vi "gfitsio-read-image-subset-i32-2d.vi"(4 "lpixel (-1,-1: rest)":cluster{"X":i32, "Y":i32}={"X"=-1, "Y"=-1}, 6 "fpixel (1,1)":cluster{"X":i32, "Y":i32}={"X"=1, "Y"=1}, 7 "inc (1,1)":cluster{"X":i32, "Y":i32}={"X"=1, "Y"=1}, 8 "error in (no error)":errorcluster, 9 "nulval (0: don't check)":i32, 11 "gfits refnum":T1) -> (0 "error out":errorcluster, 1 "anynul":bool, 2 "data":i32[][](array[numeric]), 3 "dup gfits refnum":T1)   [LabVIEW 2019, in "gfitsio.lvlib"]
doc: "Read a rectangular subimage (or the whole image) from the FITS data array. <B>fpixel</B> and <B>lpixel</B> give the coordinates of the first (lower left corner) and last (upper right corner) pixels to be read from the FITS image. Undefined FITS array elements will be set equal to <B>nullval</B> unless <B>nulval</B> is zero in which case no checks for undefined pixels will be performed."
uses:
  gfitsio.lvlib
  gfitsio-refnum.ctl
  cfitsio-hdutypes.ctl
  gfitsio.dll
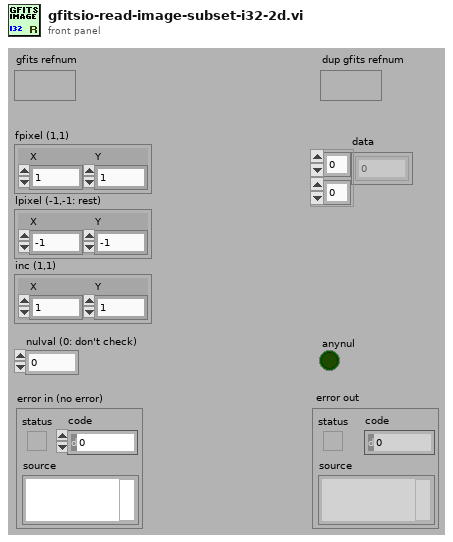
[diagram p1: front panel]
types:
  T1 = typedef "gfitsio.lvlib/gfitsio-refnum.ctl" = refnum<k1>
  T2 = typedef "gfitsio.lvlib/cfitsio-hdutypes.ctl" = i32
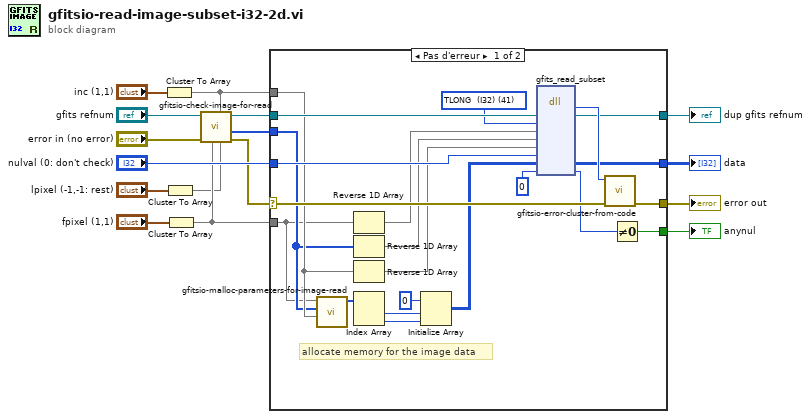
[diagram p0: block diagram]
diagram:
  n1 = Cluster To Array(cluster="inc (1,1)") -> (array=w1:i32[])
  n2 = Cluster To Array(cluster="lpixel (-1,-1: rest)") -> (array=w2:i32[])
  n3 = Cluster To Array(cluster="fpixel (1,1)") -> (array=w3:i32[])
  n4 = call "gfitsio-check-image-for-read.vi"("lpixel"=w2, "inc"=w1, "fpixel"=w3, "error in (no error)"="error in (no error)", "gfits refnum"="gfits refnum") -> ("error out"=w5:errorcluster, "lpixel out"=w4:i32[], "dup gfits refnum"=w10:T1)  [unwired: 4 in]
  n5 = case shown="Pas d'erreur" w5 {
    selector: w5 -> [w33 w39]
    tunnel: [w37 w39] -> w15
    tunnel: w10 -> [w35 w40]
    tunnel: [w34 w40] -> w16
    tunnel: "nulval (0: don't check)" -> [w32 _]
    tunnel: [w30 _] -> w13
    tunnel: [w29 _] -> w12
    tunnel: w3 -> [w22 _]
    tunnel: w4 -> [w23 _]
    tunnel: w1 -> [w24 _]
    frame No Error {
      w28 = T2 41 items=["TBIT"=1, "TBYTE  (U8)"=11, "TSBYTE  (I8)"=12, "TLOGICAL"=14, "TSTRING"=16, "TUSHORT  (U16)"=20, "TSHORT  (I16)"=21, "TUINT"=31, "TULONG  (U32)"=40, "TLONG  (I32)"=41, "TFLOAT  (SGL)"=42, "TLONGLONG  (I64)"=81, "TDOUBLE  (DBL)"=82, "TCOMPLEX  (CSG)"=83, "TDOUBLECOMPLEX  (CDB)"=163] ("cfitsio datatype")
      # "allocate memory for the image data"
      n6 = call "gfitsio-malloc-parameters-for-image-read.vi"("inc"=w24, "lpixel"=w23, "fpixel"=w22) -> ("image dimensions"=w19:i32[])  [unwired: 8 in]
      n7 = Reverse 1D Array(array=w22) -> (reversed array=w25:i32[])
      n8 = Reverse 1D Array(array=w23) -> (reversed array=w26:i32[])
      n9 = Reverse 1D Array(array=w24) -> (reversed array=w27:i32[])
      n10 = Index Array(array=w19) -> (element #1=w18:i32, element #2=w17:i32)  [unwired: 2 in]
      n11 = Initialize Array(0 ("element"), w18, w17) -> (w20:i32[][])
      n12 = dll-call lib="C:/BonOMM_git/SubVIs/gfitsio/gfitsio.dll" fn="gfits_read_subset"("dup gfits refnum"=w35, "datatype"=w28, "fpixel"=w25, "lpixel"=w26, "inc"=w27, "nulval"=w32, "array"=w20, "anynul"=0) -> (w38:i32, "dup gfits refnum"=w34:T1, "array"=w29:i32[][], "anynul"=w31:i32)  [unwired: 8 in, 2 out]
      n13 = call "gfitsio-error-cluster-from-code.vi"("error in (no error)"=w33, "error code"=w38) -> ("error out"=w37:errorcluster)  [unwired: 9 in]
      n14 = Not Equal To 0?(x=w31) -> (x != 0?=w30:bool)
    }
    frame Error {
    }
  }
  "dup gfits refnum" <- w16
  "error out" <- w15
  "anynul" <- w13
  "data" <- w12
